vi "Test Calibration wobble.vi"() -> ()   [LabVIEW 2013, in "GP22_TDC_Arduinoed.lvlib"]
uses:
  GP22_TDC_Arduinoed.lvlib
  <vilib>/Utility/file.llb/Write To Spreadsheet File (DBL).vi
  <vilib>/Analysis/NI_AALBase.lvlib
panel:
  in  "Wait time (ms)":u32=100
  out "Progress":u8(slide) scale=0.0..100.0
  in  "Output?":bool
  in  "Number of calibration readings":i32=750
  out "Histogram":dynamicdata(graph)
  out "Standard deviation":dbl format="%^_2g"
  out "Mean":dbl format="%^_2g"
  out "Calibration readings":dbl[](array[numeric])
  out "error out":errorcluster
  in  "VISA resource name":refnum<visa-resource-name>
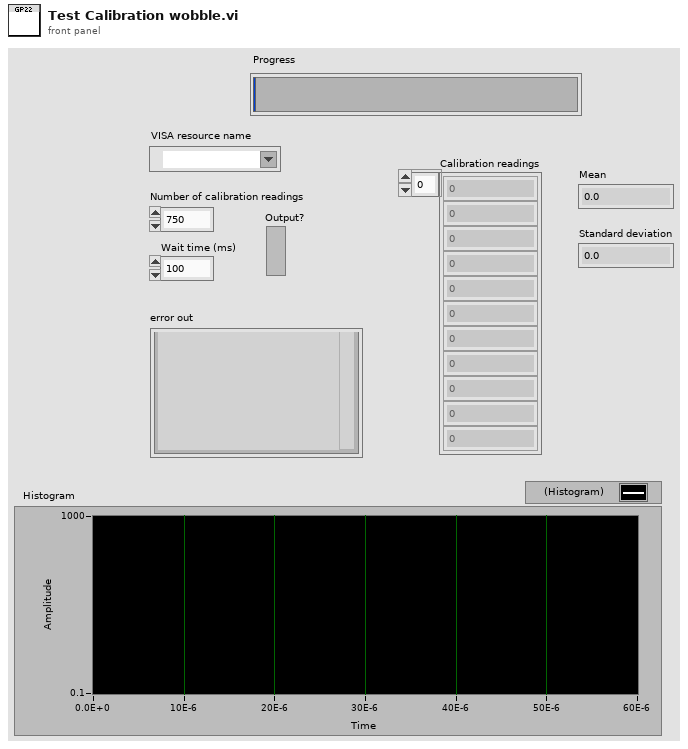
[diagram p1: front panel]
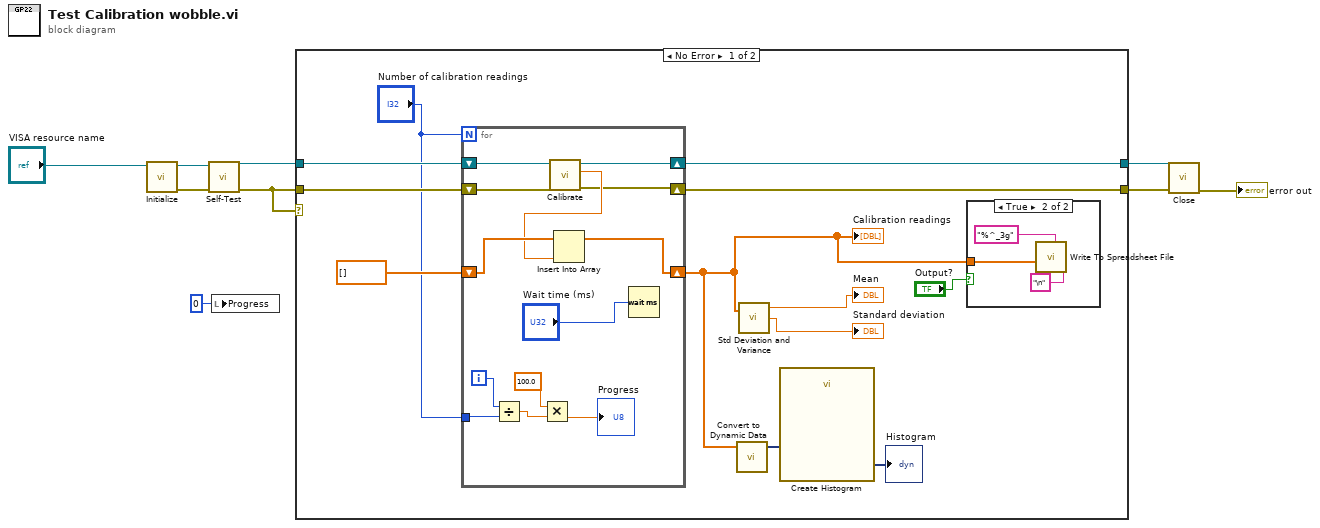
[diagram p0: block diagram]
diagram:
  n1 = call "Initialize.vi"("VISA resource name"="VISA resource name") -> ("error out"=w7:errorcluster, "VISA resource name out"=w8:refnum<visa-resource-name>)  [unwired: 9 in]
  n2 = call "Self-Test.vi"("error in (no error)"=w7, "VISA resource name"=w8) -> ("error out"=w2:errorcluster, "VISA resource name out"=w5:refnum<visa-resource-name>)  [unwired: 6 in, 2 out]
  n3 = local write "Progress"(u8 0 ("Progress")) -> ()
  n4 = case shown="No Error" w2 {
    tunnel: w5 -> [w21 w39]
    tunnel: w2 -> [w20 w38]
    tunnel: [w18 w38] -> w4
    tunnel: [w17 w39] -> w3
    frame No Error {
      n5 = for {
        N: "Number of calibration readings" -> [_]
        shift-right: [w33] -> w12
        shift-left: dbl[] [] -> [w34]
        shift-right: [w30] -> w18
        shift-left: w20 -> [w36]
        shift-right: [w31] -> w17
        shift-left: w21 -> [w37]
        tunnel: "Number of calibration readings" -> [w27]
        i -> [w28]
        n6 = Divide(x=w28, y=w27) -> (x/y=w29:dbl)
        n7 = Multiply(x=100.0, y=w29) -> (x*y=→"Progress":dbl)
        n8 = call "Calibrate.vi"("error in (no error)"=w36, "VISA resource name"=w37) -> ("error out"=w30:errorcluster, "output / s"=w32:dbl, "VISA resource name out"=w31:refnum<visa-resource-name>)  [unwired: 5 in, 1 out]
        n9 = Insert Into Array(array=w34, new element=w32) -> (w33:dbl[])  [unwired: 1 in]
        n10 = Wait (ms)(milliseconds to wait="Wait time (ms)") -> ()  [unwired: 1 out]
      }
      "Calibration readings" <- w12
      n11 = call "Convert to Dynamic Data"("Array"=w12) -> ("Dynamic Data Type"=w14:dynamicdata)  [unwired: 3 in]
      n12 = call <vilib>:"Std Deviation and Variance.vi"("X"=w12) -> ("mean"=→"Mean":dbl, "standard deviation"=→"Standard deviation":dbl)  [unwired: 1 in, 1 out]
      n13 = call "Create Histogram"("Signal"=w14) -> ("Histogram"=→"Histogram":dynamicdata)  [unwired: 9 in, 1 out]
      n14 = case shown="True" "Output?" {
        tunnel: w12 -> [_ w24]
        frame False {
        }
        frame True {
          n15 = call-poly <vilib>:"Write To Spreadsheet File.vi"("delimiter (\\t)"="\n" ("delimiter (\\t)"), "format (%.3f)"="%^_3g", "1D data"=w24) -> ()  [unwired: 5 in, 1 out]
        }
      }
    }
    frame Error {
    }
  }
  n16 = call "Close.vi"("error in (no error)"=w4, "VISA resource name"=w3) -> ("error out"=→"error out":errorcluster)  [unwired: 9 in]
